vi "Initialize.vi"(6 "Set Defaults? (F)":bool, 7 "Serial Configuration":T1={"Baud Rate"=9600, "Parity"=0, "Data Bits"=8, "Stop Bits"=10, "Flow Control"=0} {"Flow Control" items=["None", "XON/XOFF", "RTS/CTS", "XON/XOFF & RTS/CTS", "DTR/DSR", "XON/XOFF & DTR/DSR"]; "Stop Bits" items=["1.0"=10, "1.5"=15, "2.0"=20]; "Data Bits" items=["7"=7, "8"=8]; "Parity" items=["None", "Odd", "Even", "Mark", "Space"]; "Baud Rate" items=["300"=300, "600"=600, "1200"=1200, "2400"=2400, "4800"=4800, "9600"=9600, "19200"=19200]}, 8 "error in (no error)":errorcluster, 9 "Reset (True)":bool=TRUE, 10 "ID Query (True)":bool=TRUE, 11 "VISA resource name":refnum<visa-resource-name>) -> (0 "error out":errorcluster, 3 "VISA resource name out":refnum<visa-resource-name>)   [LabVIEW 2011, in "MGC647C.lvlib"]
doc: "Establishes communication with the instrument and optionally performs an instrument identification query and/or an instrument reset. It also places the instrument in a default state needed for other instrument driver operations. Therefore, call this VI before calling other instrument driver VIs for this instrument. Generally, you need to call the Initialize VI only once at the beginning of an application."
uses:
  <instrlib>/MGC647C/MGC647C.lvlib
panel:
  # "(C) Copyright 2012 GSI Helmholtzzentrum für Schwerionenforschung GmbH.  ALL RIGHTS RESERVED."
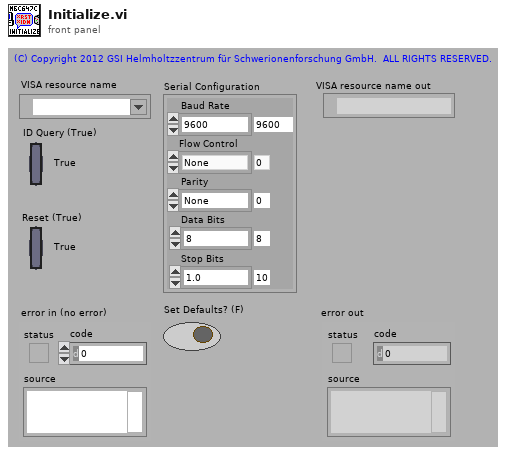
[diagram p1: front panel]
types:
  T1 = cluster{"Baud Rate":u32, "Parity":u16, "Data Bits":u16, "Stop Bits":u16, "Flow Control":u16}
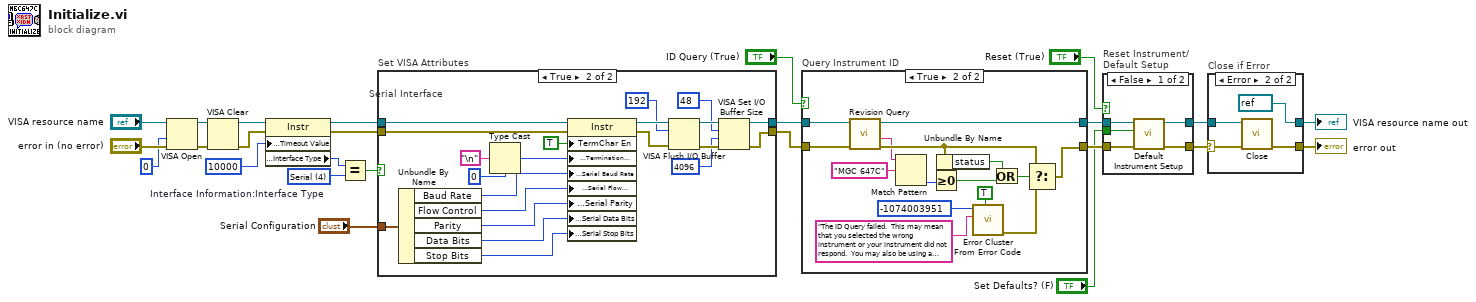
[diagram p0: block diagram]
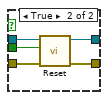
[diagram p4: hidden frame]
diagram:
  w12 = u16 4 items=["GPIB"=1, "VXI"=2, "GPIB-VXI"=3, "Serial"=4, "PXI"=5, "TCPIP"=6, "USB"=7]  # Interface Information:Interface Type
  n1 = VISA Open(access mode=u32 0, error in (no error)="error in (no error)", VISA resource name="VISA resource name") -> (VISA resource name=w10:refnum<visa-resource-name>, error out=w9:errorcluster)  [unwired: 2 in]
  n2 = VISA Clear(VISA resource name=w10, error in (no error)=w9) -> (VISA resource name out=w8:refnum<visa-resource-name>, error out=w7:errorcluster)
  n3 = property class="Instr"(reference=w8, error in=w7, "General Settings:Timeout Value"=u32 10000) -> (reference out=w15:refnum<visa-resource-name>, error out=w14:errorcluster, "Interface Information:Interface Type"=w19:u16)
  n4 = Equal?(x=w19, y=w12) -> (x = y?=w13:bool)
  n5 = case "Set VISA Attributes" shown="True" w13 {
    tunnel: [w26 w45] -> w17
    tunnel: [w27 w42] -> w16
    tunnel: w15 -> [w26 w47]
    tunnel: w14 -> [w27 w48]
    tunnel: "Serial Configuration" -> [_ w28]
    frame False {
      # "TCP/IP"
    }
    frame True {
      # "Serial Interface"
      n6 = Unbundle By Name(w28) -> ("Baud Rate"=w34:u32, "Flow Control"=w31:u16, "Parity"=w32:u16, "Data Bits"=w33:u16, "Stop Bits"=w30:u16)
      n7 = Type Cast(type=u8 0, x="\n" ("Line Feed Constant")) -> (*(type *) &x=w35:u8)
      n8 = property class="Instr"(reference=w47, error in=w48, "TermChar En"=TRUE ("Message Based Settings:Termination Character Enable"), "Message Based Settings:Termination Character"=w35, "Serial Settings:Serial Baud Rate"=w34, "Serial Settings:Serial Flow Control"=w31, "Serial Settings:Serial Parity"=w32, "Serial Settings:Serial Data Bits"=w33, "Serial Settings:Serial Stop Bits"=w30) -> (reference out=w41:refnum<visa-resource-name>, error out=w44:errorcluster)
      n9 = VISA Flush I/O Buffer(VISA resource name=w41, mask (16)=u16 192, error in (no error)=w44) -> (VISA resource name out=w46:refnum<visa-resource-name>, error out=w43:errorcluster)
      n10 = VISA Set I/O Buffer Size(VISA resource name=w46, mask (16)=u16 48, size (4096)=u32 4096 ("size (0)"), error in (no error)=w43) -> (VISA resource name out=w45:refnum<visa-resource-name>, error out=w42:errorcluster)
    }
  }
  n11 = case "Query Instrument ID" shown="True" "ID Query (True)" {
    tunnel: [w49 w65] -> w24
    tunnel: [w50 w54] -> w25
    tunnel: w17 -> [w50 w55]
    tunnel: w16 -> [w49 w53]
    frame False {
    }
    frame True {
      n12 = call <instrlib>:"Revision Query.vi"("error in (no error)"=w53, "VISA resource name"=w55) -> ("error out"=w52:errorcluster, "Instrument Firmware Revision"=w51:string, "VISA resource name out"=w54:refnum<visa-resource-name>)  [unwired: 6 in, 1 out]
      n13 = Match Pattern(string=w51, regular expression="MGC 647C") -> (offset past match=w59:i32)  [unwired: 1 in, 3 out]
      n14 = Greater Or Equal To 0?(x=w59) -> (x >= 0?=w57:bool)
      n15 = Unbundle By Name(w52) -> ("status"=w58:bool)
      n16 = call <vilib>:"Error Cluster From Error Code.vi"("show call chain? (False)"=TRUE, "error message (\"\")"="The ID Query failed.  This may mean that you selected the wrong instrument or your instrument did not respond.  You may also be using a model that is not officially supported by this driver.  If you are sure that you have selected the correct instrument and it is responding, try disabling the ID Query." ("Source (VI Name)"), "error code (0)"=-1074003951 ("Code")) -> ("error out"=w63:errorcluster)  [unwired: 6 in]
      n17 = Or(x=w58, y=w57) -> (x .or. y?=w56:bool)
      n18 = Select(t=w52, s=w56, f=w63) -> (s? t:f=w65:errorcluster)
    }
  }
  n19 = case "Reset Instrument/\nDefault Setup" shown="False" "Reset (True)" {
    tunnel: w24 -> [w69 w72]
    tunnel: [w67 w75] -> w3
    tunnel: w25 -> [w70 w73]
    tunnel: [w68 w74] -> w4
    tunnel: "Set Defaults? (F)" -> [w66 w71]
    frame False {
      n20 = call <instrlib>:"Default Instrument Setup.vi"("error in (no error)"=w69, "Set Defaults? (F)"=w66, "VISA resource name"=w70) -> ("error out"=w67:errorcluster, "VISA resource name out"=w68:refnum<visa-resource-name>)  [unwired: 7 in]
    }
    frame True {
      n21 = call <instrlib>:"Reset.vi"("error in (no error)"=w72, "Set Defaults? (F)"=w71, "VISA resource name"=w73) -> ("error out"=w75:errorcluster, "VISA resource name out"=w74:refnum<visa-resource-name>)  [unwired: 7 in]
    }
  }
  n22 = case "Close if Error" shown="Error" w3 {
    selector: w3 -> [w76 w79]
    tunnel: w4 -> [w77 w80]
    tunnel: [w77 refnum<visa-resource-name> refnum ("VISA resource name out")] -> w6
    tunnel: [w76 w81] -> w5
    frame No Error {
    }
    frame Error {
      n23 = call <instrlib>:"Close.vi"("error in (no error)"=w79, "VISA resource name"=w80) -> ("error out"=w81:errorcluster)  [unwired: 9 in]
    }
  }
  "VISA resource name out" <- w6
  "error out" <- w5
